vi "Select Channel Dialog.vi"(6 "Item Names":string[][](array[string]), 7 "DisplayFilter":u8(ring)=7 items=["K_CHAN_R", "K_CHAN_W", "K_CHAN_RW", "K_CHAN_VOLT", "K_CHAN_FAULT", "K_ALL", "K_CUSTOM", "K_CHAN_R_VIS", "K_CHAN_W_VIS", "K_CHAN_RW_VIS", "K_CHAN_VOLT_VIS", "K_CHAN_FAULT_VIS"], 8 "error in (no error)":errorcluster, 9 "Caption":string, 10 "nodePath":string, 11 "NIVS.System Definition Root":refnum<k24>) -> (0 "error out":errorcluster, 1 "Caption out":string, 2 "Cancel?":bool, 3 "Selected Item":T2, 4 "Item Names":string[][](array[string]))   [LabVIEW 2013, in "CANopen Workspace Objects.lvlib"]
uses:
  CANopen Workspace Objects.lvlib
  NationalInstruments.VeriStand.SystemStorageUI
  NationalInstruments.VeriStand.SystemStorage
  <vilib>/NI Veristand/UI Controls/Single Node Browser/Node Ref.ctl
  NationalInstruments.VeriStand
  <vilib>/NI Veristand/UI Controls/Single Node Browser/NI_VS UI Single Node Browser.lvlib
panel:
  in  "CANopen sets":T1(ring)
  in  "Cancel":bool
  in  "OK":bool
  in  "Value":i64
  in  "Name":string
  in  "Text Value Pairing":i32(listbox)
  in  "Single Node Browser":refnum<k24>(container)
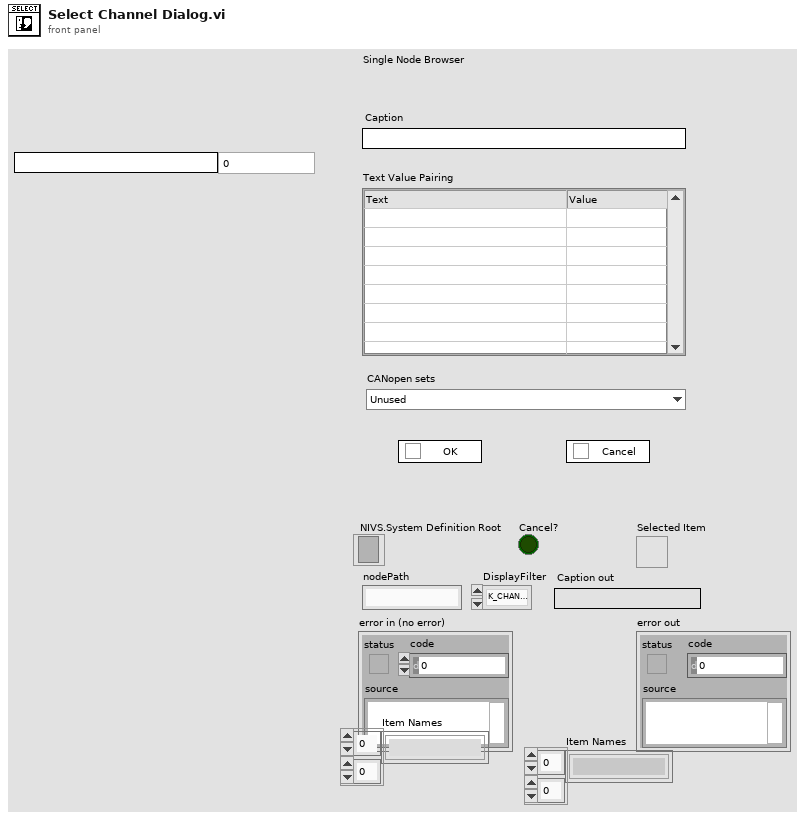
[diagram p1: front panel]
types:
  T1 = enum16{"Unused", "Device state", "NMT command", "Byte Order", "Data Type"}
  T2 = typedef "NI_VS UI Single Node Browser.lvlib/Node Ref.ctl" = refnum<k24>
  T3 = typedef "NI_VS UI Single Node Browser.lvlib/Callback Type.ctl" = cluster{"Net Callbacks":refnum<k27>[], "Event":refnum<user-event>}
  T4 = typedef "LVPoint32TypeDef.ctl" = cluster{"Horizontal":i32, "Vertical":i32}
  T5 = typedef "LVRowAndColumnTypeDef.ctl" = cluster{"Row":i32, "Column":i32}
  T6 = typedef "LVPositionTypeDef.ctl" = cluster{"Left":i32, "Top":i32}
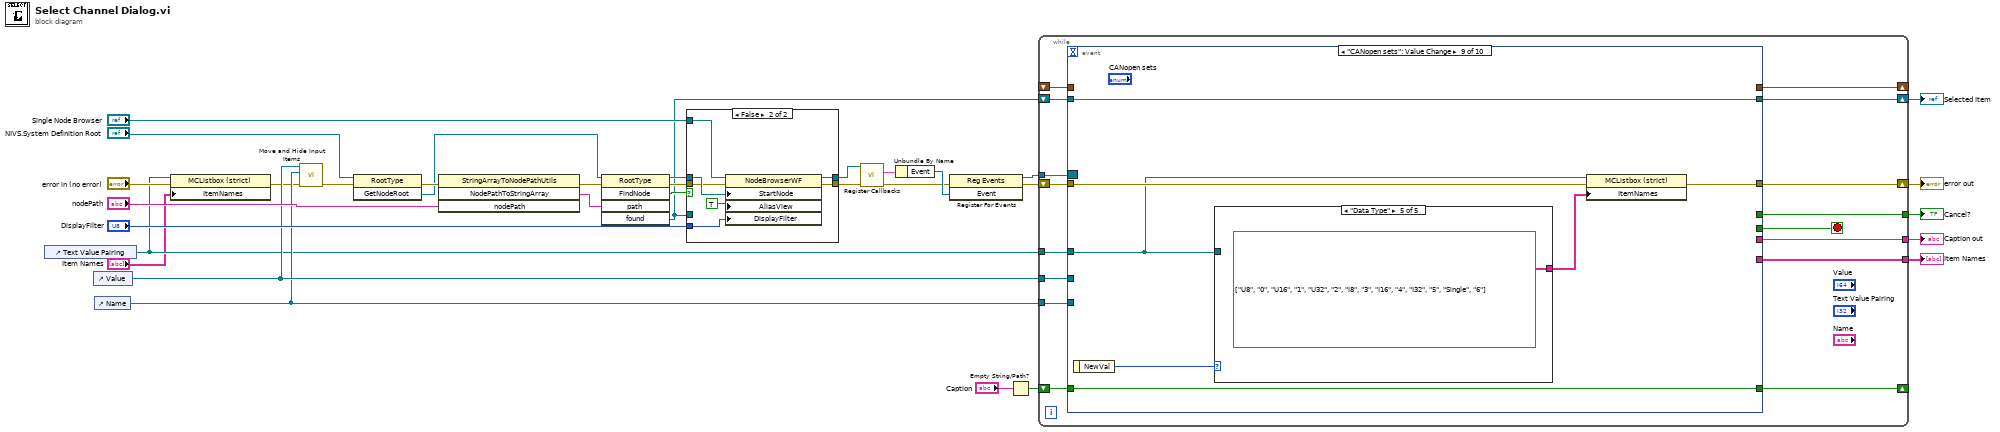
[diagram p0: block diagram]
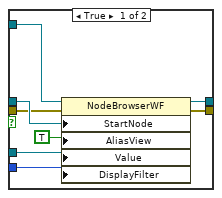
[diagram p2: hidden frame]
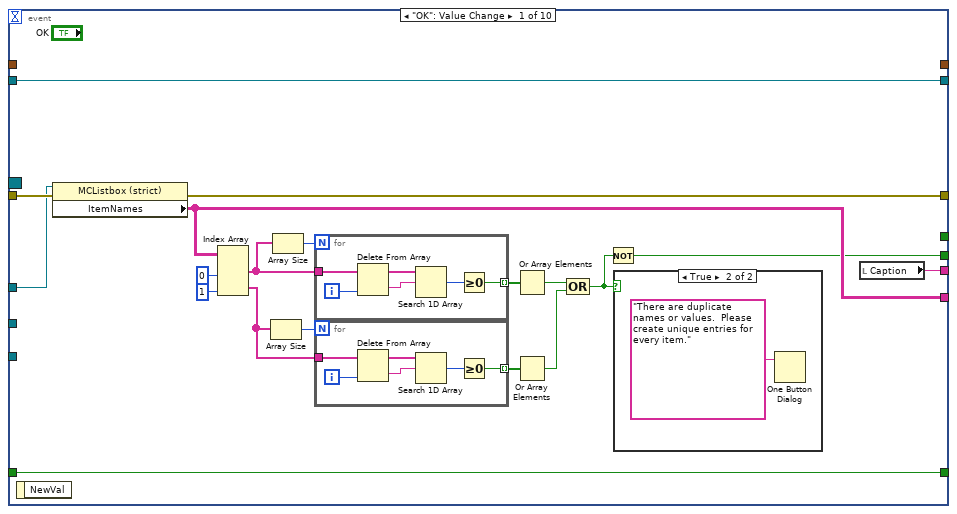
[diagram p3: hidden frame]
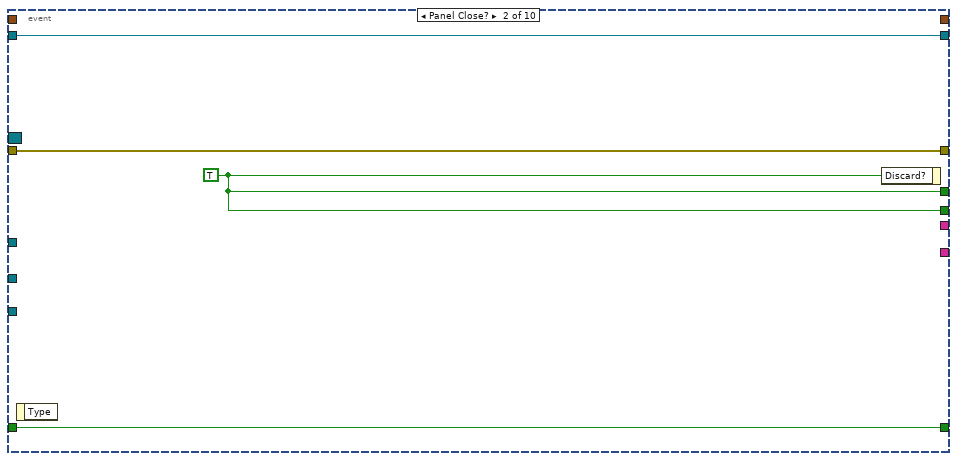
[diagram p5: hidden frame]
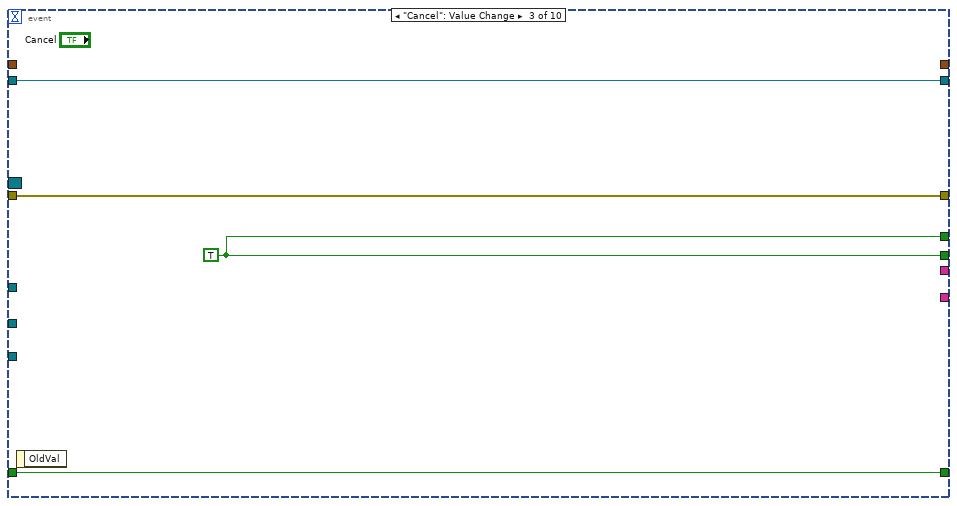
[diagram p6: hidden frame]
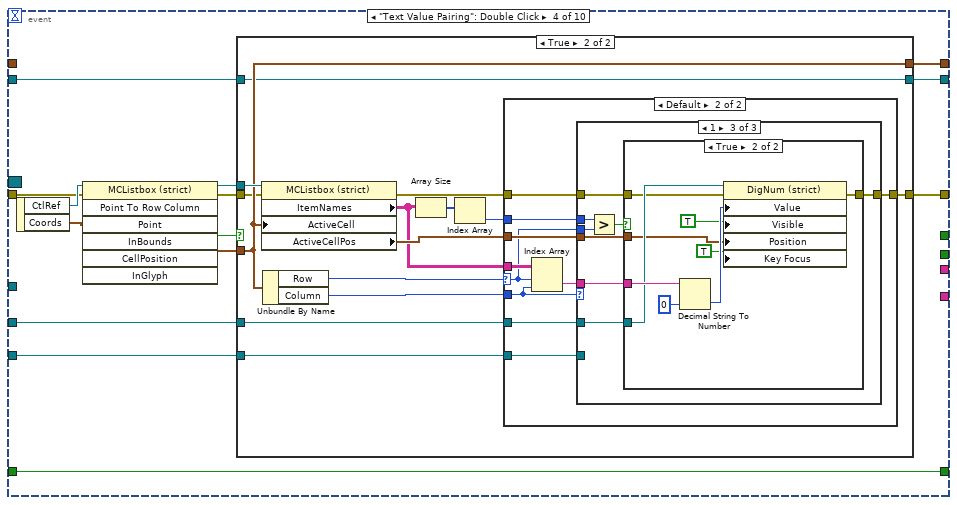
[diagram p7: hidden frame]
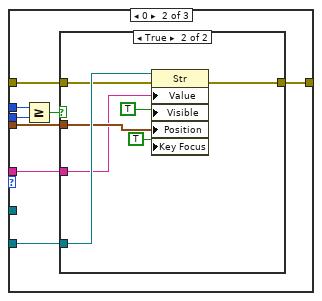
[diagram p11: hidden frame]
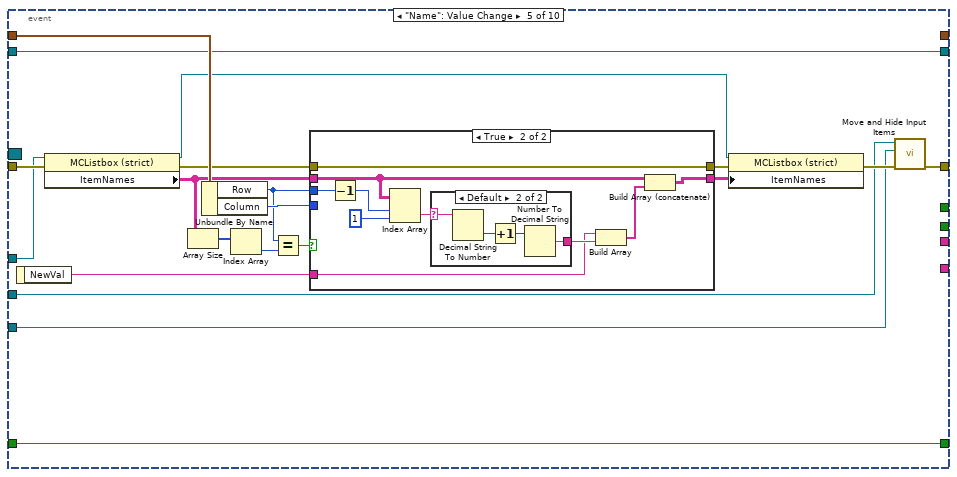
[diagram p14: hidden frame]
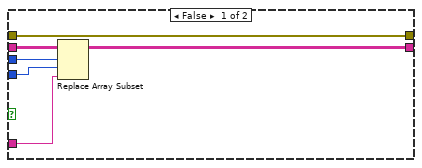
[diagram p15: hidden frame]
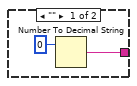
[diagram p16: hidden frame]
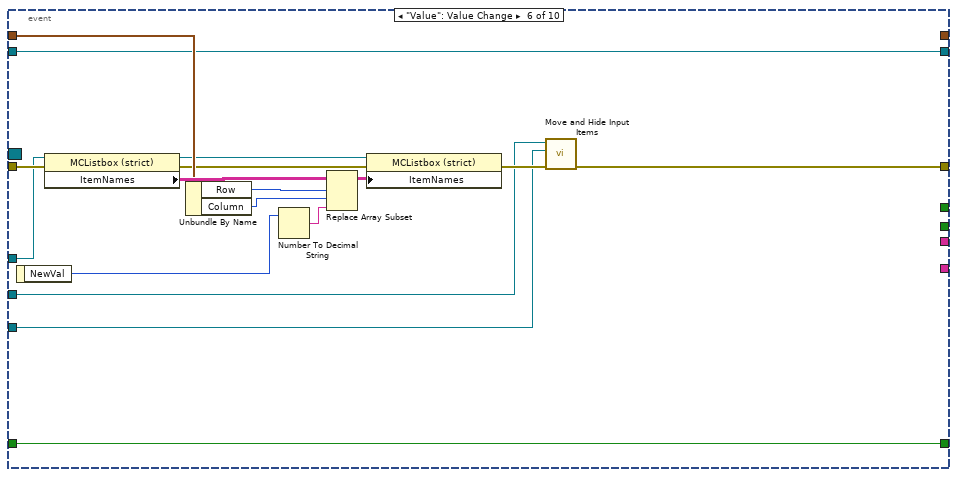
[diagram p17: hidden frame]
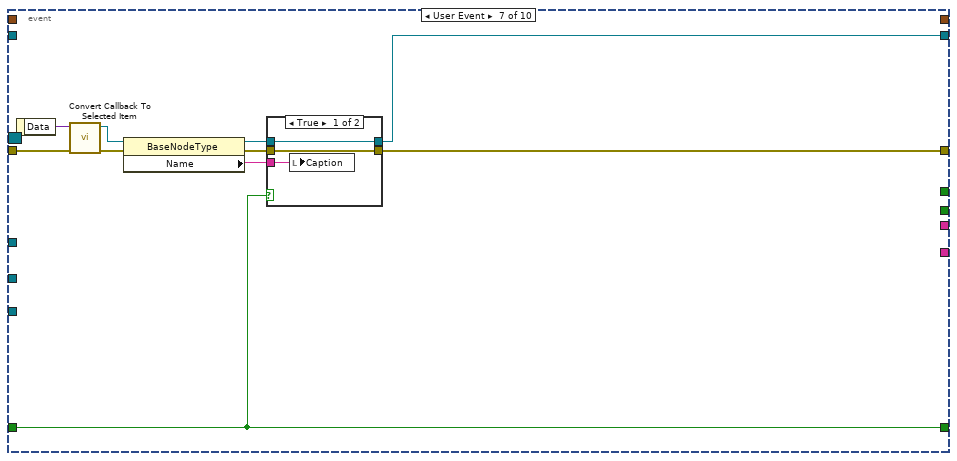
[diagram p18: hidden frame]
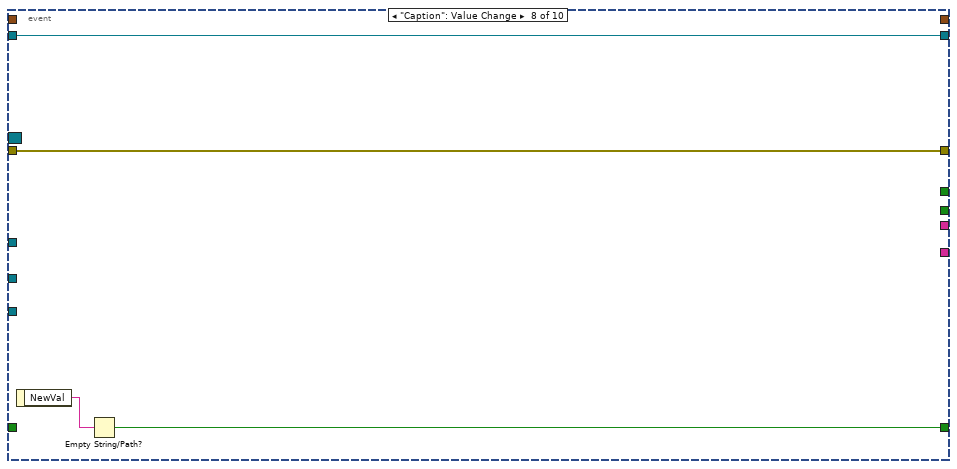
[diagram p20: hidden frame]
diagram:
  n1 = control-ref of="Text Value Pairing"() -> (w5:refnum<vi>)
  n2 = control-ref of="Value"() -> (w12:refnum<vi>)
  n3 = control-ref of="Name"() -> (w11:refnum<vi>)
  n4 = property class="MCListbox (strict)"(reference=w5, error in="error in (no error)", "ItemNames"="Item Names") -> (error out=w6:errorcluster)  [unwired: 1 out]
  n5 = call "Move and Hide Input Items.vi"("error in (no error)"=w6, "Name"=w11, "Value"=w12) -> ("error out"=w10:errorcluster)  [unwired: 8 in]
  n6 = invoke class="RootType" method="GetNodeRoot"(reference="NIVS.System Definition Root", error in=w10) -> (error out=w25:errorcluster, "GetNodeRoot"=w23:refnum<k24>)  [unwired: 1 in, 1 out]
  n7 = invoke class="StringArrayToNodePathUtils" method="NodePathToStringArray"(error in=w25, "nodePath"="nodePath") -> (error out=w24:errorcluster, "NodePathToStringArray"=w26:string[])  [unwired: 2 in, 2 out]
  n8 = invoke class="RootType" method="FindNode"(reference=w23, error in=w24, "path"=w26) -> (reference out=w17:refnum<k24>, error out=w27:errorcluster, "FindNode"=w21:bool, "found"=w1:refnum<k24>)  [unwired: 2 in, 1 out]
  n9 = case shown="False" w21 {
    tunnel: "DisplayFilter" -> [w36 w42]
    tunnel: "Single Node Browser" -> [w41 w48]
    tunnel: [w40 w47] -> w20
    tunnel: w17 -> [w39 w46]
    tunnel: w27 -> [w38 w45]
    tunnel: w1 -> [w37 _]
    tunnel: [w34 w44] -> w15
    frame True {
      n10 = property class="NodeBrowserWF"(reference=w41, error in=w38, "StartNode"=w39, "AliasView"=TRUE, "Value"=w37, "DisplayFilter"=w36) -> (reference out=w34:refnum<k24>, error out=w40:errorcluster)
    }
    frame False {
      n11 = property class="NodeBrowserWF"(reference=w48, error in=w45, "StartNode"=w46, "AliasView"=TRUE, "DisplayFilter"=w42) -> (reference out=w44:refnum<k24>, error out=w47:errorcluster)
    }
  }
  n12 = call <vilib>:"Register Callbacks.vi"("error in (no error)"=w20, "Single Node Browser"=w15) -> ("error out"=w19:errorcluster, "Callbacks"=w33:T3)  [unwired: 7 in, 1 out]
  n13 = Unbundle By Name(w33) -> ("Event"=w32:refnum<user-event>)
  n14 = register-events(error in=w19, w32) -> (reference out=w13:refnum<event-registration>, error out=w18:errorcluster)  [unwired: 1 in]
  n15 = Empty String/Path?(string/path="Caption") -> (empty?=w2:bool)
  n16 = while {
    tunnel: w13 -> [w64]
    shift-right: [w62] -> w30
    shift-left: w18 -> [w61]
    tunnel: [w60] -> w29
    shift-right: [w59] -> w14
    shift-left: w1 -> [w58]
    shift-right: [w57] -> _
    shift-left: _ -> [w56]
    tunnel: w12 -> [w55]
    tunnel: w11 -> [w54]
    tunnel: [w53] -> w9
    tunnel: w5 -> [w52]
    tunnel: [w51] -> w8
    shift-right: [w49] -> _
    shift-left: w2 -> [w50]
    stop <- w63 stop-if-true
    n17 = event shown="[8] \"CANopen sets\": Value Change" {
      selector: w64 -> [_ _ _ _ _ _ _ _ _ _]
      dyn-events: _ -> [_ _ _ _ _ _ _ _ _ _]
      timeout: _ -> [_ _ _ _ _ _ _ _ _ _]
      tunnel: [w65 w100 w104 _ _ _ _ _ _ _] -> w63
      tunnel: w61 -> [w82 w97 w101 w106 w200 w239 w248 w255 w263 w272]
      tunnel: [w81 w97 w101 w107 w190 w227 w240 w255 w262 w275] -> w62
      tunnel: [_ w100 w104 _ _ _ _ _ _ _] -> w60
      tunnel: [w83 w99 w103 w109 w189 w226 w243 w258 w265 w277] -> w59
      tunnel: w58 -> [w83 w99 w103 w108 w189 w226 _ w258 w265 w277]
      tunnel: w55 -> [_ _ _ w113 w192 w225 _ _ _ w274]
      tunnel: w54 -> [_ _ _ w112 w191 w224 _ _ _ w273]
      tunnel: [_ _ _ w111 _ _ _ _ _ w278] -> w57
      tunnel: w56 -> [_ _ _ _ w197 w235 _ _ _ w278]
      tunnel: w52 -> [w80 _ _ _ w199 w238 _ _ w260 _]
      tunnel: [w79 _ _ _ _ _ _ _ _ _] -> w53
      tunnel: [w71 _ _ _ _ _ _ _ _ _] -> w51
      tunnel: w50 -> [w78 w98 w102 w105 w188 w223 w241 _ w264 w276]
      tunnel: [w78 w98 w102 w105 w188 w223 w241 w256 w264 w276] -> w49
      event "OK": Value Change {
        n18 = event-data() -> ()  [unwired: 1 in, 1 out]
        n19 = property class="MCListbox (strict)"(reference=w80, error in=w82) -> (error out=w81:errorcluster, "ItemNames"=w71:string[][])  [unwired: 1 out]
        n20 = Index Array(array=w71, index (col) #1=0 ("disabled index (col)"), index (col) #2=1 ("index (col)")) -> (element #1=w74:string[], element #2=w69:string[])  [unwired: 2 in]
        n21 = Array Size(array=w69) -> (size(s)=w70:i32)
        n22 = Array Size(array=w74) -> (size(s)=w75:i32)
        n23 = for {
          N: w75 -> [_]
          tunnel: w74 -> [w96]
          tunnel: [w91] -> w73 mode=indexing
          i -> [w95]
          n24 = Delete From Array(array=w96, index=w95) -> (deleted portion=w93:string, array with subset deleted=w94:string[])  [unwired: 1 in]
          n25 = Search 1D Array(1D array=w94, element=w93) -> (index of element=w92:i32)  [unwired: 1 in]
          n26 = Greater Or Equal To 0?(x=w92) -> (x >= 0?=w91:bool)
        }
        n27 = for {
          N: w70 -> [_]
          tunnel: w69 -> [w90]
          tunnel: [w85] -> w68 mode=indexing
          i -> [w89]
          n28 = Delete From Array(array=w90, index=w89) -> (deleted portion=w87:string, array with subset deleted=w88:string[])  [unwired: 1 in]
          n29 = Search 1D Array(1D array=w88, element=w87) -> (index of element=w86:i32)  [unwired: 1 in]
          n30 = Greater Or Equal To 0?(x=w86) -> (x >= 0?=w85:bool)
        }
        n31 = Or Array Elements(Boolean array=w73) -> (logical OR=w72:bool)
        n32 = Or Array Elements(Boolean array=w68) -> (logical OR=w67:bool)
        n33 = Compound Arithmetic op=OR(w72, w67) -> (w66:bool)
        n34 = Not(x=w66) -> (.not. x?=w65:bool)
        n35 = case shown="True" w66 {
          frame False {
          }
          frame True {
            n36 = One Button Dialog(message="There are duplicate names or values.  Please create unique entries for every item.") -> ()  [unwired: 1 in, 1 out]
          }
        }
        n37 = local read "Caption"() -> (w79:string)
      }
      event Panel Close? {
        w100 = TRUE ("Discard?")
        n38 = event-data() -> ()  [unwired: 1 in, 1 out]
        n39 = event-data("Discard?"=w100) -> ()  [unwired: 1 in, 1 out]
      }
      event "Cancel": Value Change {
        w104 = TRUE ("Discard?")
        n40 = event-data() -> ()  [unwired: 1 in, 1 out]
      }
      event "Text Value Pairing": Double Click {
        n41 = event-data() -> ("CtlRef"=w118:refnum<vi>, "Coords"=w117:T4)  [unwired: 1 in]
        n42 = invoke class="MCListbox (strict)" method="Point To Row Column"(reference=w118, error in=w106, "Point"=w117) -> (reference out=w116:refnum<vi>, error out=w110:errorcluster, "InBounds"=w114:bool, "CellPosition"=w115:T5)  [unwired: 4 in, 3 out]
        n43 = case shown="True" w114 {
          tunnel: w115 -> [_ w130]
          tunnel: w116 -> [_ w134]
          tunnel: w113 -> [_ w133]
          tunnel: w112 -> [_ w131]
          tunnel: [_ w130] -> w111
          tunnel: w110 -> [w119 w128]
          tunnel: [w120 w129] -> w109
          tunnel: w108 -> [w120 w129]
          tunnel: [w119 w126] -> w107
          frame False {
          }
          frame True {
            n44 = property class="MCListbox (strict)"(reference=w134, error in=w128, "ActiveCell"=w130) -> (error out=w127:errorcluster, "ItemNames"=w125:string[][], "ActiveCellPos"=w132:T6)  [unwired: 1 out]
            n45 = Unbundle By Name(w130) -> ("Row"=w121:i32, "Column"=w123:i32)
            n46 = Array Size(array=w125) -> (size(s)=w124:i32[])
            n47 = Index Array(array=w124) -> (element=w122:i32)  [unwired: 1 in]
            n48 = case shown="Default" w121 {
              selector: w121 -> [_ w136]
              tunnel: w133 -> [_ w144]
              tunnel: w132 -> [_ w143]
              tunnel: w131 -> [_ w142]
              tunnel: w127 -> [w135 w141]
              tunnel: [w135 w140] -> w126
              tunnel: w125 -> [_ w139]
              tunnel: w123 -> [_ w138]
              tunnel: w122 -> [_ w137]
              frame -1 {
              }
              frame Default {
                n49 = Index Array(array=w139, index (row)=w136, index (col)=w138) -> (element=w145:string)
                n50 = case shown="1" w138 {
                  tunnel: w145 -> [_ w152 w170]
                  tunnel: w143 -> [_ w153 w168]
                  tunnel: w144 -> [_ _ w169]
                  tunnel: w142 -> [_ w154 _]
                  tunnel: w141 -> [w146 w151 w167]
                  tunnel: [w146 w150 w166] -> w140
                  tunnel: w137 -> [_ w149 w165]
                  tunnel: w136 -> [_ w148 w164]
                  frame Default {
                  }
                  frame 0 {
                    n51 = Greater Or Equal?(x=w149, y=w148) -> (x >= y?=w147:bool)
                    n52 = case shown="True" w147 {
                      tunnel: w154 -> [_ w162]
                      tunnel: w153 -> [_ w161]
                      tunnel: w152 -> [_ w160]
                      tunnel: w151 -> [w155 w158]
                      tunnel: [w155 w156] -> w150
                      frame False {
                      }
                      frame True {
                        n53 = property class="Str"(reference=w162, error in=w158, "Value"=w160, "Visible"=TRUE, "Position"=w161, "Key Focus"=TRUE) -> (error out=w156:errorcluster)  [unwired: 1 out]
                      }
                    }
                  }
                  frame 1 {
                    n54 = Greater?(x=w165, y=w164) -> (0:w163:bool)
                    n55 = case shown="True" w163 {
                      tunnel: w170 -> [_ w180]
                      tunnel: w169 -> [_ w179]
                      tunnel: w168 -> [_ w176]
                      tunnel: w167 -> [w171 w174]
                      tunnel: [w171 w172] -> w166
                      frame False {
                      }
                      frame True {
                        n56 = Decimal String To Number(string=w180, default (0L)=i64 0 ("default (0 I32)")) -> (number=w178:i64)  [unwired: 1 in, 1 out]
                        n57 = property class="DigNum (strict)"(reference=w179, error in=w174, "Value"=w178, "Visible"=TRUE, "Position"=w176, "Key Focus"=TRUE) -> (error out=w172:errorcluster)  [unwired: 1 out]
                      }
                    }
                  }
                }
              }
            }
          }
        }
      }
      event "Name": Value Change {
        n58 = event-data() -> ("NewVal"=w198:string)  [unwired: 1 in]
        n59 = property class="MCListbox (strict)"(reference=w199, error in=w200) -> (reference out=w194:refnum<vi>, error out=w181:errorcluster, "ItemNames"=w185:string[][])
        n60 = Array Size(array=w185) -> (size(s)=w187:i32[])
        n61 = Unbundle By Name(w197) -> ("Row"=w184:i32, "Column"=w196:i32)
        n62 = Index Array(array=w187) -> (element=w186:i32)  [unwired: 1 in]
        n63 = Equal?(x=w184, y=w186) -> (x = y?=w183:bool)
        n64 = case shown="True" w183 {
          tunnel: w198 -> [w206 w209]
          tunnel: w196 -> [w205 _]
          tunnel: [w204 w216] -> w195
          tunnel: w185 -> [w203 w215]
          tunnel: w184 -> [w202 w214]
          tunnel: [w201 w208] -> w182
          tunnel: w181 -> [w201 w208]
          frame False {
            n65 = Replace Array Subset(array=w203, new element=w206, index (row)=w202, index (col)=w205) -> (w204:string[][])
          }
          frame True {
            n66 = Decrement(x=w214) -> (x-1=w213:i32)
            n67 = Index Array(array=w215, index (row)=w213, index (col)=1 ("disabled index (col)")) -> (element=w211:string)
            n68 = case shown="Default" w211 {
              selector: w211 -> [_ w220]
              tunnel: [w217 w219] -> w210
              frame "" {
                n69 = Number To Decimal String(number=0) -> (decimal integer string=w217:string)  [unwired: 1 in]
              }
              frame Default {
                n70 = Decimal String To Number(string=w220) -> (number=w221:i32)  [unwired: 2 in, 1 out]
                n71 = Increment(x=w221) -> (x+1=w222:i32)
                n72 = Number To Decimal String(number=w222) -> (decimal integer string=w219:string)  [unwired: 1 in]
              }
            }
            n73 = Build Array(w209, w210) -> (w207:string[])
            n74 = Build Array (concatenate)(w215, w207) -> (w216:string[][])
          }
        }
        n75 = property class="MCListbox (strict)"(reference=w194, error in=w182, "ItemNames"=w195) -> (error out=w193:errorcluster)  [unwired: 1 out]
        n76 = call "Move and Hide Input Items.vi"("error in (no error)"=w193, "Name"=w191, "Value"=w192) -> ("error out"=w190:errorcluster)  [unwired: 8 in]
      }
      event "Value": Value Change {
        n77 = event-data() -> ("NewVal"=w236:i64)  [unwired: 1 in]
        n78 = property class="MCListbox (strict)"(reference=w238, error in=w239) -> (reference out=w230:refnum<vi>, error out=w232:errorcluster, "ItemNames"=w237:string[][])
        n79 = Unbundle By Name(w235) -> ("Row"=w234:i32, "Column"=w233:i32)
        n80 = Number To Decimal String(number=w236) -> (decimal integer string=w229:string)  [unwired: 1 in]
        n81 = Replace Array Subset(array=w237, new element=w229, index (row)=w234, index (col)=w233) -> (w231:string[][])
        n82 = property class="MCListbox (strict)"(reference=w230, error in=w232, "ItemNames"=w231) -> (error out=w228:errorcluster)  [unwired: 1 out]
        n83 = call "Move and Hide Input Items.vi"("error in (no error)"=w228, "Name"=w224, "Value"=w225) -> ("error out"=w227:errorcluster)  [unwired: 8 in]
      }
      event User Event {
        n84 = event-data() -> ("Data"=w249:variant)  [unwired: 1 in]
        n85 = call <vilib>:"Convert Callback To Selected Item.vi"("error in"=w248, "Data"=w249) -> ("error out"=w246:errorcluster, "Selected Item"=w247:T2)  [unwired: 8 in]
        n86 = property class="BaseNodeType"(reference=w247, error in=w246) -> (reference out=w242:T2, error out=w244:errorcluster, "Name"=w245:string)
        n87 = case shown="True" w241 {
          tunnel: w245 -> [w252 _]
          tunnel: [w251 w254] -> w240
          tunnel: w244 -> [w251 w254]
          tunnel: [w250 w253] -> w243
          tunnel: w242 -> [w250 w253]
          frame True {
            n88 = local write "Caption"(w252) -> ()
          }
          frame False {
          }
        }
      }
      event "Caption": Value Change {
        n89 = event-data() -> ("NewVal"=w257:string)  [unwired: 1 in]
        n90 = Empty String/Path?(string/path=w257) -> (empty?=w256:bool)
      }
      event "CANopen sets": Value Change {
        n91 = event-data() -> ("NewVal"=w261:T1)  [unwired: 1 in]
        n92 = case shown="\"Data Type\"" w261 {
          tunnel: w260 -> [w267 _ _ _ _]
          tunnel: [w266 string[][] [["unknown", "1"], ["bootup", "0"], ["stopped", "4"], ["operational", "5"], ["preoperational", "127"], ["connection lost", "128"]] ("ItemNames") string[][] [["idle", "0"], ["start remote node", "1"], ["stop remote node", "2"], ["enter pre-operational", "3"], ["reset node", "4"], ["reset communication from node side", "5"], ["reinit communication from NI VS side", "6"]] ("ItemNames") string[][] [["big-endian, network order", "0"], ["little-endian", "1"]] ("ItemNames") string[][] [["U8", "0"], ["U16", "1"], ["U32", "2"], ["I8", "3"], ["I16", "4"], ["I32", "5"], ["Single", "6"]] ("ItemNames")] -> w259
          frame "Unused", Default {
            n93 = property class="MCListbox (strict)"(reference=w267) -> ("ItemNames"=w266:string[][])  [unwired: 1 in, 2 out]
          }
          frame "Device state" {
          }
          frame "NMT command" {
          }
          frame "Byte Order" {
          }
          frame "Data Type" {
          }
        }
        n94 = property class="MCListbox (strict)"(reference=w260, error in=w263, "ItemNames"=w259) -> (error out=w262:errorcluster)  [unwired: 1 out]
      }
      event "Value", "Name": Mouse Leave {
        n95 = event-data() -> ()  [unwired: 1 in, 1 out]
        n96 = call "Move and Hide Input Items.vi"("error in (no error)"=w272, "Name"=w273, "Value"=w274) -> ("error out"=w275:errorcluster)  [unwired: 8 in]
      }
    }
  }
  "error out" <- w30
  "Cancel?" <- w29
  "Caption out" <- w9
  "Item Names" <- w8
  "Selected Item" <- w14
